vi "Write Display - Form.vi"(8 "error in (no error)":errorcluster, 10 "form":T1, 11 "NT Scalar (Numeric) in":refnum<class "NT Scalar (Numeric).lvclass">) -> (0 "error out":errorcluster, 3 "NT Scalar (Numeric) out":refnum<class "NT Scalar (Numeric).lvclass">)   [LabVIEW 2020, in "PV Access.lvlib" / "PV Data.lvlib" / "NT Scalar (Numeric).lvclass"]
uses:
  NT Scalar (Numeric).lvclass
  NT Scalar (Numeric).lvclass/NT Scalar (Numeric).ctl
  Display Form.ctl
  PV Data.lvlib
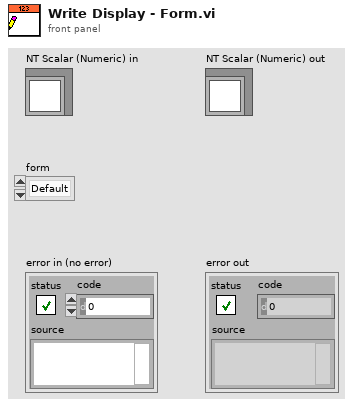
[diagram p1: front panel]
types:
  T1 = typedef "PV Access.lvlib/PV Data.lvlib/Display Form.ctl" = enum16{"Default", "String", "Binary", "Decimal", "Hex", "Exponential", "Engineering"}
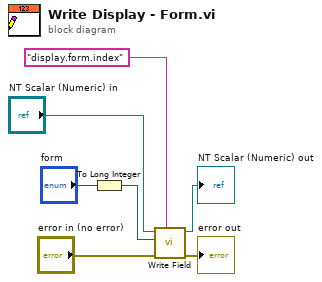
[diagram p0: block diagram]
diagram:
  n1 = To Long Integer(number="form") -> (32bit integer=w2:i32)
  n2 = call-dynamic "Write Field.vi"("field"="display.form.index", "error in (no error)"="error in (no error)", "value"=w2, "Base Interface in"="NT Scalar (Numeric) in") -> ("error out"=→"error out":errorcluster, "Base Interface out"=→"NT Scalar (Numeric) out":refnum<class "NT Scalar (Numeric).lvclass">)  [unwired: 6 in]
